vi "Get Scan Info.vi"(11 "String Input":string="$AGENT.81,C8.C8,S*03") -> (0 "溫度":string, 1 "壓力":string, 2 "OK and NG":bool, 3 "晶片ID":string, 4 "雷雕ID":string)   [LabVIEW 2019]
panel:
  out "before substring":string
  out "after substring 3":string
  out "OK and NG":string
  out "after substring":string
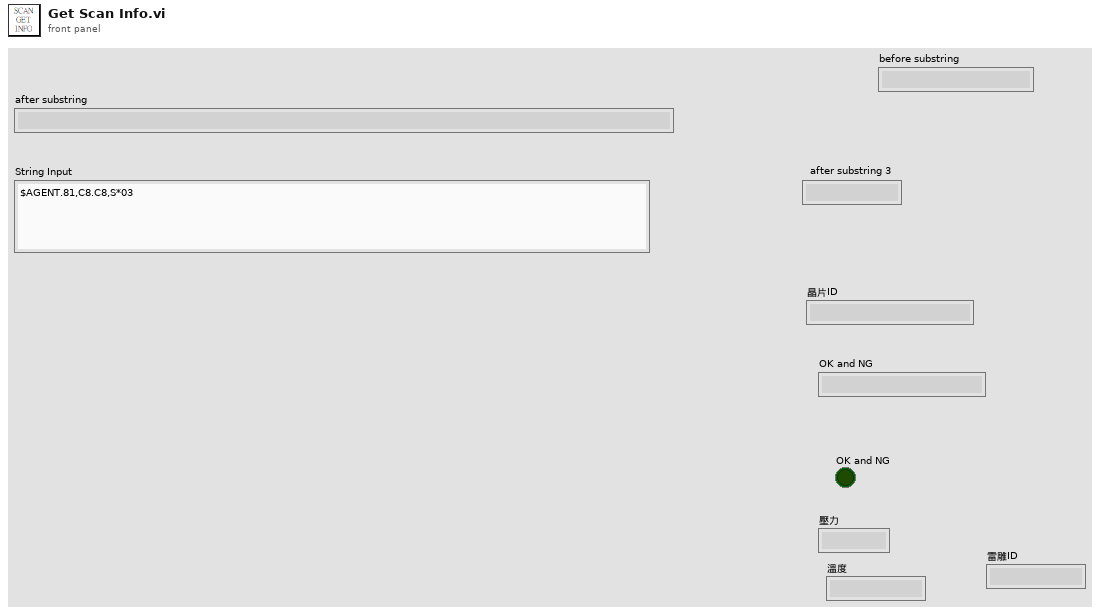
[diagram p1: front panel]
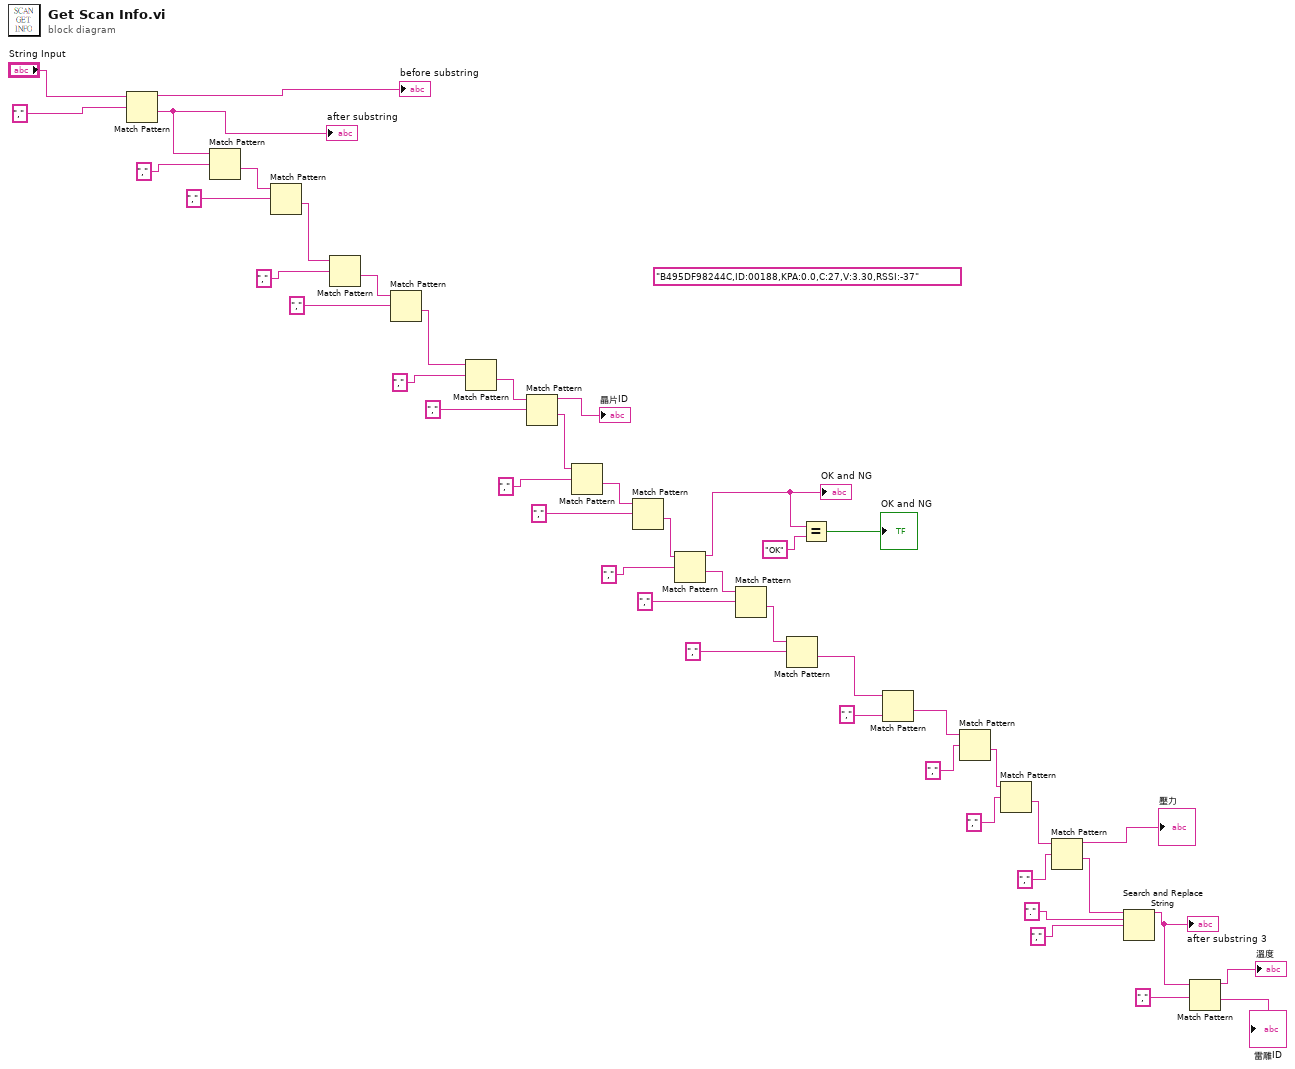
[diagram p0: block diagram]
diagram:
  (unwired) "B495DF98244C,ID:00188,KPA:0.0,C:27,V:3.30,RSSI:-37"
  n1 = Match Pattern(string="String Input", regular expression=",") -> (before substring=→"before substring":string, after substring=w44:string)  [unwired: 1 in, 2 out]
  "after substring" <- w44
  n2 = Match Pattern(string=w44, regular expression=",") -> (after substring=w43:string)  [unwired: 1 in, 3 out]
  n3 = Match Pattern(string=w43, regular expression=",") -> (after substring=w24:string)  [unwired: 1 in, 3 out]
  n4 = Match Pattern(string=w24, regular expression=",") -> (after substring=w39:string)  [unwired: 1 in, 3 out]
  n5 = Match Pattern(string=w39, regular expression=",") -> (after substring=w27:string)  [unwired: 1 in, 3 out]
  n6 = Match Pattern(string=w27, regular expression=",") -> (after substring=w36:string)  [unwired: 1 in, 3 out]
  n7 = Match Pattern(string=w36, regular expression=",") -> (before substring=→"晶片ID":string, after substring=w18:string)  [unwired: 1 in, 2 out]
  n8 = Match Pattern(string=w18, regular expression=",") -> (after substring=w33:string)  [unwired: 1 in, 3 out]
  n9 = Match Pattern(string=w33, regular expression=",") -> (after substring=w26:string)  [unwired: 1 in, 3 out]
  n10 = Match Pattern(string=w26, regular expression=",") -> (before substring=w16:string, after substring=w30:string)  [unwired: 1 in, 2 out]
  "OK and NG" <- w16
  n11 = Match Pattern(string=w30, regular expression=",") -> (after substring=w25:string)  [unwired: 1 in, 3 out]
  n12 = Match Pattern(string=w25, regular expression=",") -> (after substring=w22:string)  [unwired: 1 in, 3 out]
  n13 = Equal?(x=w16, y="OK") -> (x = y?=→"OK and NG":bool)
  n14 = Match Pattern(string=w22, regular expression=",") -> (after substring=w21:string)  [unwired: 1 in, 3 out]
  n15 = Match Pattern(string=w21, regular expression=",") -> (after substring=w12:string)  [unwired: 1 in, 3 out]
  n16 = Match Pattern(string=w12, regular expression=",") -> (after substring=w10:string)  [unwired: 1 in, 3 out]
  n17 = Match Pattern(string=w10, regular expression=",") -> (before substring=→"壓力":string, after substring=w6:string)  [unwired: 1 in, 2 out]
  n18 = Search and Replace String(input string=w6, search string=".", replace string=",") -> (result string=w5:string)  [unwired: 5 in, 3 out]
  "after substring 3" <- w5
  n19 = Match Pattern(string=w5, regular expression=",") -> (before substring=→"溫度":string, after substring=→"雷雕ID":string)  [unwired: 1 in, 2 out]
